vi "Rapid Read_5Ch_VR2.vi"(0 "Dig Cards":refnum<k15>[](array[refnum]), 3 "Channel":string="1", 5 "Motion Board ID":T1=1 min=1 max=32 step=1, 9 "rf points per line":i32, 11 "error in":errorcluster, 12 "lines per plane":i32, 13 "queue out":refnum<queue>) -> (6 "Reverse?":bool, 10 "Dig Word Size":u16, 15 "error out":errorcluster)   [LabVIEW 2022 SP3]
uses:
  Motion Controllers/-MotionRoutines/MotionGlobals.vi
  <instrlib>/niScope/Acquire/Fetch/niScope Multi Fetch Binary 8.vi
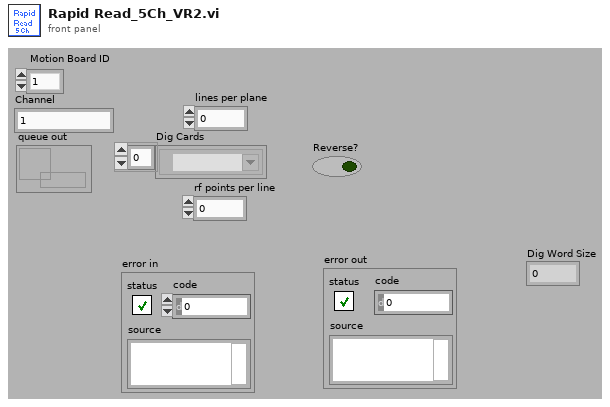
[diagram p1: front panel]
types:
  T1 = typedef "Board Id" = u8
  T2 = cluster{"Dig Cards[0]":refnum<k15>, "Dig Cards[1]":refnum<k15>, "Dig Cards[2]":refnum<k15>, "Dig Cards[3]":refnum<k15>, "Dig Cards[4]":refnum<k15>}
  T3 = typedef "Var" = u8
  T4 = cluster{"actualSamples":i32, "absoluteInitialX":dbl, "relativeInitialX":dbl, "xIncrement":dbl, "offset":dbl, "gain":dbl, "reserved1":dbl, "reserved2":dbl}[]
  T5 = cluster{"actualSamples":i32, "absoluteInitialX":dbl, "relativeInitialX":dbl, "xIncrement":dbl, "offset":dbl, "gain":dbl, "reserved1":dbl, "reserved2":dbl}
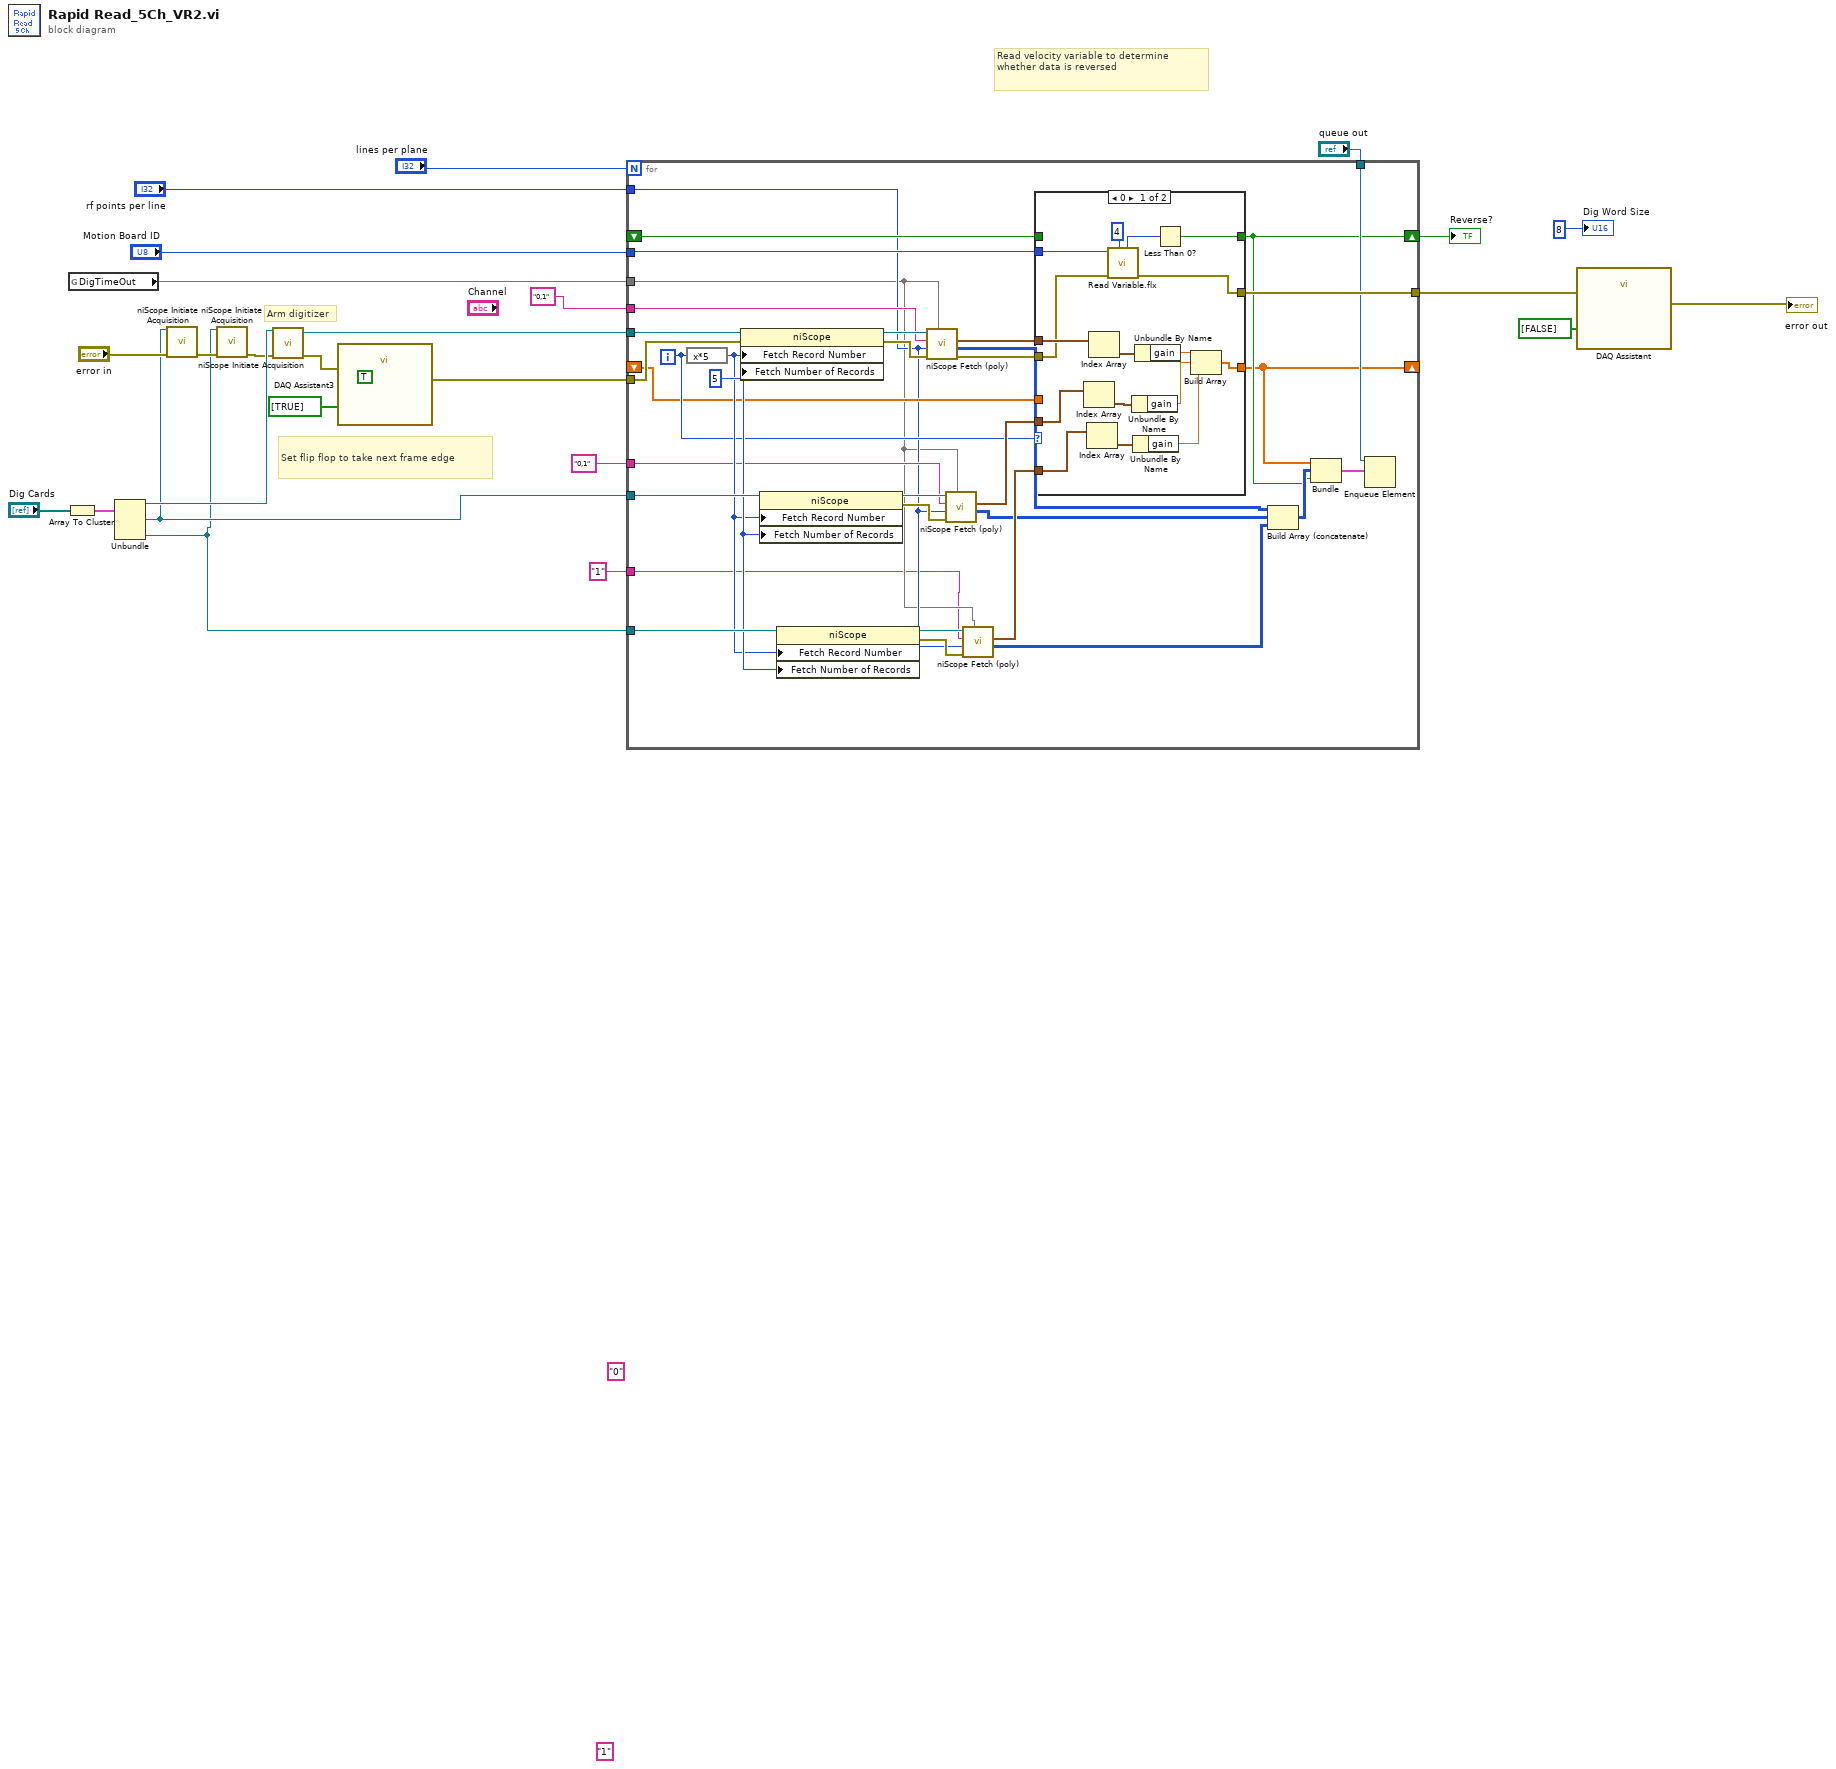
[diagram p0: block diagram]
diagram:
  (unwired) "1" ("Channel")
  (unwired) "0" ("Channel")
  (unwired) TRUE ("stop (T)")
  # "Set flip flop to take next frame edge"
  # "Arm digitizer"
  # "Read velocity variable to determine whether data is reversed"
  n1 = Array To Cluster(array="Dig Cards") -> (cluster=w17:T2)
  n2 = global read "MotionGlobals.vi" "DigTimeOut"() -> (w14)
  n3 = Unbundle(w17) -> ("Dig Cards[0]"=w11:refnum<k15>, "Dig Cards[2]"=w2:refnum<k15>, "Dig Cards[4]"=w1:refnum<k15>)  [unwired: 2 out]
  n4 = call <instrlib>:"niScope Initiate Acquisition.vi"("instrument handle"=w2, "error in"="error in") -> ("error out"=w10:errorcluster)  [unwired: 1 in, 12 out]
  n5 = call <instrlib>:"niScope Initiate Acquisition.vi"("instrument handle"=w1, "error in"=w10) -> ("error out"=w8:errorcluster)  [unwired: 1 in, 12 out]
  n6 = call <instrlib>:"niScope Initiate Acquisition.vi"("instrument handle"=w11, "error in"=w8) -> ("instrument handle out"=w22:refnum<k15>, "error out"=w19:errorcluster)  [unwired: 1 in, 11 out]
  n7 = call "DAQ Assistant3"("data"=bool[] [TRUE], "error in"=w19) -> ("error out"=w7:errorcluster)  [unwired: 2 in, 15 out]
  n8 = for {
    N: "lines per plane" -> [_]
    tunnel: "Motion Board ID" -> [w59]
    tunnel: "rf points per line" -> [w28]
    tunnel: w14 -> [w27]
    tunnel: w22 -> [w58]
    tunnel: w7 -> [w57]
    tunnel: "0,1" ("Channel") -> [w52]
    tunnel: [w51] -> w16
    tunnel: w2 -> [w44]
    tunnel: w1 -> [w43]
    tunnel: "0,1" ("Channel") -> [w40]
    shift-right: [w30] -> _
    shift-left: _ -> [w38]
    shift-right: [w31] -> w15
    shift-left: _ -> [w37]
    tunnel: "queue out" -> [w32]
    tunnel: "1" ("Channel") -> [w26]
    i -> [w39]
    w42 = 5
    n9 = expression code="x*5"(w39) -> (w41:i32)
    n10 = property class="niScope"(reference=w58, error in=w57, "Fetch Record Number"=w41, "Fetch Number of Records"=w42) -> (reference out=w56:refnum<k15>, error out=w55:errorcluster)
    n11 = property class="niScope"(reference=w44, "Fetch Record Number"=w41, "Fetch Number of Records"=w42) -> (reference out=w50:refnum<k15>, error out=w49:errorcluster)  [unwired: 1 in]
    n12 = property class="niScope"(reference=w43, "Fetch Record Number"=w41, "Fetch Number of Records"=w42) -> (reference out=w47:refnum<k15>, error out=w46:errorcluster)  [unwired: 1 in]
    n13 = call-poly <instrlib>:"niScope Fetch (poly).vi"("timeout"=w27, "error in"=w55, "numSamples"=w28, "channels"=w52, "instrument handle"=w56) -> ("error out"=w53:errorcluster, "wfm"=w36:i8[][], "wfm info"=w54:T4)  [unwired: 4 out]
    n14 = call-poly <instrlib>:"niScope Fetch (poly).vi"("timeout"=w27, "error in"=w49, "numSamples"=w28, "channels"=w40, "instrument handle"=w50) -> ("wfm"=w35:i8[][], "wfm info"=w48:T4)  [unwired: 5 out]
    n15 = call-poly <instrlib>:"niScope Fetch (poly).vi"("timeout"=w27, "error in"=w46, "numSamples"=w28, "channels"=w26, "instrument handle"=w47) -> ("wfm"=w34:i8[][], "wfm info"=w45:T4)  [unwired: 5 out]
    n16 = case shown="0" w39 {
      tunnel: w59 -> [w75 _]
      tunnel: w54 -> [w74 _]
      tunnel: w53 -> [w73 w77]
      tunnel: [w69 w76] -> w31
      tunnel: [w68 w77] -> w51
      tunnel: w48 -> [w67 _]
      tunnel: w45 -> [w65 _]
      tunnel: [w60 w78] -> w30
      tunnel: w38 -> [_ w78]
      tunnel: w37 -> [_ w76]
      frame 0 {
        n17 = Index Array(array=w67) -> (element=w66:T5)  [unwired: 1 in]
        n18 = Index Array(array=w65) -> (element=w64:T5)  [unwired: 1 in]
        n19 = Index Array(array=w74) -> (element=w70:T5)  [unwired: 1 in]
        n20 = call <vilib>:"Read Variable.flx"("Var"=T3 4, "error in (no error)"=w73, "Board ID"=w75) -> ("error out"=w68:errorcluster, "Output"=w71:i32)  [unwired: 1 in, 4 out]
        n21 = Unbundle By Name(w66) -> ("gain"=w62:dbl)
        n22 = Unbundle By Name(w64) -> ("gain"=w61:dbl)
        n23 = Unbundle By Name(w70) -> ("gain"=w63:dbl)
        n24 = Less Than 0?(x=w71) -> (x < 0?=w69:bool)
        n25 = Build Array(w63, w62, w61) -> (w60:dbl[])
      }
      frame 1, Default {
      }
    }
    n26 = Build Array (concatenate)(w36, w35, w34) -> (w33:i8[][])
    n27 = Bundle(w30, w33, w31) -> (w29:cluster{dbl[], i8[][], bool})  [unwired: 1 in]
    n28 = Enqueue Element(queue=w32, element=w29) -> ()  [unwired: 2 in, 3 out]
  }
  "Reverse?" <- w15
  n29 = call "DAQ Assistant"("data"=bool[] [FALSE], "error in"=w16) -> ("error out"=→"error out":errorcluster)  [unwired: 2 in, 15 out]
  "Dig Word Size" <- 8
